vi "CoreCommand.vi"(8 "error in (no error)":errorcluster, 9 "Data":variant, 10 "Msg":T1, 11 "Module_Interface in":refnum<class "Module_Interface.lvclass">) -> (0 "error out":errorcluster, 3 "Module_Interface out":refnum<class "Module_Interface.lvclass">)   [LabVIEW 2025, in "Module.lvlib" / "Module_Interface.lvclass"]
uses:
  Module_Interface.lvclass
  Msg.ctl
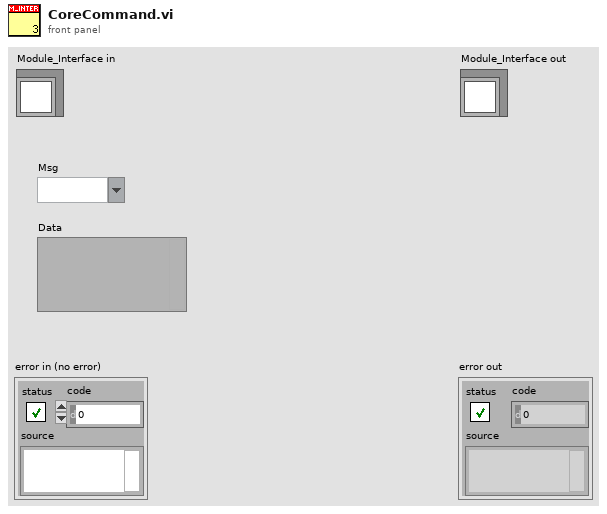
[diagram p1: front panel]
types:
  T1 = typedef "Msg.ctl" = string
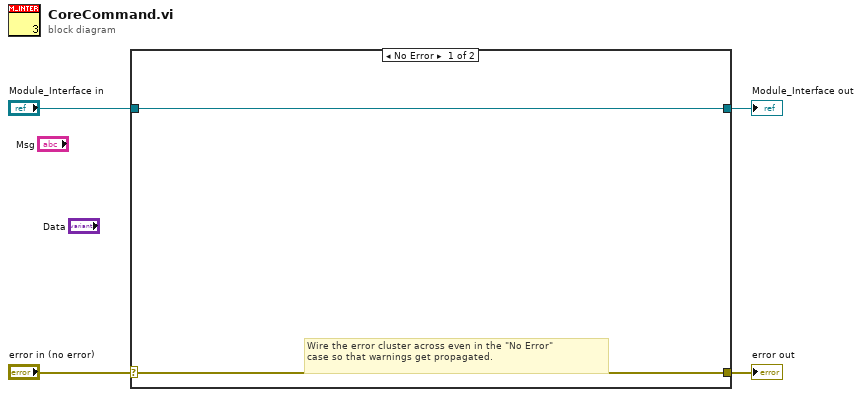
[diagram p0: block diagram]
diagram:
  n1 = case shown="No Error" "error in (no error)" {
    selector: "error in (no error)" -> [w6 w8]
    tunnel: [w6 w8] -> w3
    tunnel: [w5 w7] -> w1
    tunnel: "Module_Interface in" -> [w5 w7]
    frame No Error {
      # "Wire the error cluster across even in the \"No Error\"\ncase so that warnings get propagated."
    }
    frame Error {
    }
  }
  "error out" <- w3
  "Module_Interface out" <- w1
